vi "ITR HP.vi"(7 "input":dbl format="%.2f", 13 "corner period (steps)":dbl(slide)=10.237739663395852 scale=1.0..1000.0) -> (8 "output":dbl format="%.2f")   [LabVIEW 2019]
doc: "Modular ITR first order High pass filter with internal shift registers.\n\nJuan Gamez\nPhysics 350\nCSUSB Physics"
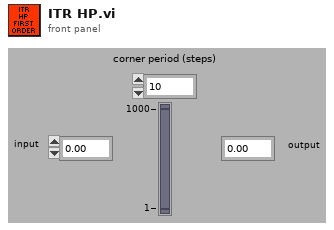
[diagram p1: front panel]
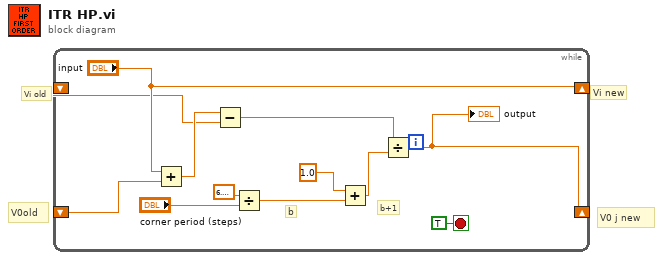
[diagram p0: block diagram]
diagram:
  # "V0old"
  # "V0 j new"
  # "Vi old"
  # "Vi new"
  n1 = while {
    shift-left: _ -> [w1]
    shift-right: ["input"] -> _
    shift-right: [w4] -> _
    shift-left: _ -> [w7]
    stop <- TRUE stop-if-true
    # "b+1"
    # "b"
    n2 = Add(x="input", y=w7) -> (x+y=w2:dbl)
    n3 = Subtract(x=w2, y=w1) -> (x-y=w5:dbl)
    n4 = Divide(x=6.283185307179586, y="corner period (steps)") -> (x/y=w8:dbl)
    n5 = Add(x=1.0, y=w8) -> (x+y=w6:dbl)
    n6 = Divide(x=w5, y=w6) -> (x/y=w4:dbl)
    "output" <- w4
  }
